vi "Version Manager.vi"(8 "error in (no error)":errorcluster, 11 "Device Item Ref In in":T1 format="%.0x") -> (0 "error out":errorcluster, 3 "Device Item Ref In out":T1 format="%.0x")   [LabVIEW 2020, in "Vires VTD System Explorer.lvlib"]
uses:
  Vires VTD System Explorer.lvlib
  <vilib>/NI VeriStand/Custom Device API/Custom Device Item Ref.ctl
  NationalInstruments.VeriStand.SystemDefinitionAPI
  <vilib>/NI VeriStand/Custom Device API/Custom Device API.lvlib
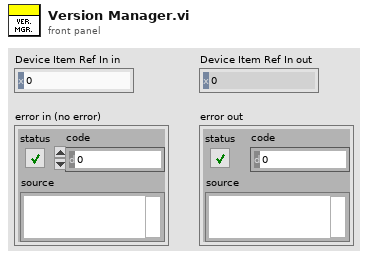
[diagram p1: front panel]
types:
  T1 = typedef "Custom Device API.lvlib/Custom Device Item Ref.ctl" = u64
  T2 = typedef "Custom Device API.lvlib/Custom Device Item Info.ctl" = cluster{"Name":string, "Is Channel":bool, "GUID":string, "Is Waveform":bool}
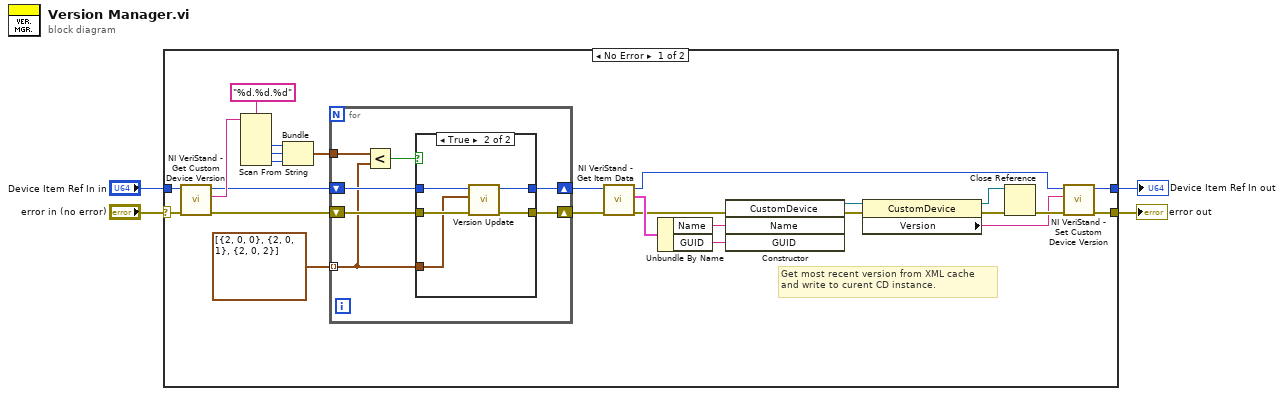
[diagram p0: block diagram]
diagram:
  n1 = case shown="No Error" "error in (no error)" {
    selector: "error in (no error)" -> [w29 w45]
    tunnel: "Device Item Ref In in" -> [w30 w46]
    tunnel: [w11 w46] -> w2
    tunnel: [w12 w45] -> w1
    frame No Error {
      # "Get most recent version from XML cache\nand write to curent CD instance."
      n2 = call <vilib>:"NI VeriStand - Get Custom Device Version.vi"("error in (no error)"=w29, "Device Ref in"=w30) -> ("error out"=w7:errorcluster, "Value"=w24:string, "Device Ref out"=w10:T1)  [unwired: 7 in]
      n3 = Scan From String(format string="%d.%d.%d", input string=w24) -> (output 1=w27:i32, output 2=w28:i32, output 3=w25:i32)  [unwired: 5 in, 3 out]
      n4 = Bundle(w27, w28, w25) -> (w6:cluster{i32, i32, i32})  [unwired: 1 in]
      n5 = for {
        tunnel: w6 -> [w37]
        tunnel: cluster{i32, i32, i32}[] [{2, 0, 0}, {2, 0, 1}, {2, 0, 2}] -> [w31] mode=indexing
        shift-right: [w35] -> w9
        shift-left: w10 -> [w34]
        shift-right: [w33] -> w8
        shift-left: w7 -> [w32]
        n6 = Less?(x=w37, y=w31) -> (x < y?=w36:bool)
        n7 = case shown="True" w36 {
          tunnel: [w39 w41] -> w35
          tunnel: w34 -> [w39 w43]
          tunnel: [w38 w42] -> w33
          tunnel: w32 -> [w38 w44]
          tunnel: w31 -> [_ w40]
          frame False {
          }
          frame True {
            n8 = call "Version Update.vi"("error in (no error)"=w44, "Version"=w40, "Device Item Ref In in"=w43) -> ("error out"=w42:errorcluster, "Device Item Ref In out"=w41:T1)  [unwired: 7 in]
          }
        }
      }
      n9 = call <vilib>:"NI VeriStand - Get Item Data.vi"("error in (no error)"=w8, "Item Ref in"=w9) -> ("error out"=w20:errorcluster, "Item Info"=w23:T2, "Item Ref out"=w13:T1)  [unwired: 6 in, 1 out]
      n10 = Unbundle By Name(w23) -> ("Name"=w22:string, "GUID"=w21:string)
      n11 = constructor class="CustomDevice"(error in=w20, "Name"=w22, "GUID"=w21) -> (reference out=w19:refnum<k24>, error out=w18:errorcluster)  [unwired: 2 in, 3 out]
      n12 = property class="CustomDevice"(reference=w19, error in=w18) -> (reference out=w16:refnum<k24>, error out=w17:errorcluster, "Version"=w14:string)
      n13 = Close Reference(reference=w16, error in (no error)=w17) -> (error out=w15:errorcluster)
      n14 = call <vilib>:"NI VeriStand - Set Custom Device Version.vi"("error in (no error)"=w15, "Value"=w14, "Device Ref in"=w13) -> ("error out"=w12:errorcluster, "Device Ref out"=w11:T1)  [unwired: 7 in]
    }
    frame Error {
    }
  }
  "error out" <- w1
  "Device Item Ref In out" <- w2
